vi "PostProcess.vi"(8 "error in (no error)":errorcluster, 10 "Variant in":variant, 11 "ONNX Angle Class in":refnum<class "ONNX Angle Class.lvclass">) -> (0 "error out":errorcluster, 2 "Variant out":variant, 3 "ONNX Angle Class out":refnum<class "ONNX Angle Class.lvclass">)   [LabVIEW 2017, in "ONNX Angle Class Library.lvlib" / "ONNX Angle Class.lvclass"]
uses:
  ONNX Angle Class.lvclass
  <vilib>/picture/picture.llb/imagedata.ctl
  ONNX Angle Class Library.lvlib
panel:
  out "image":picture
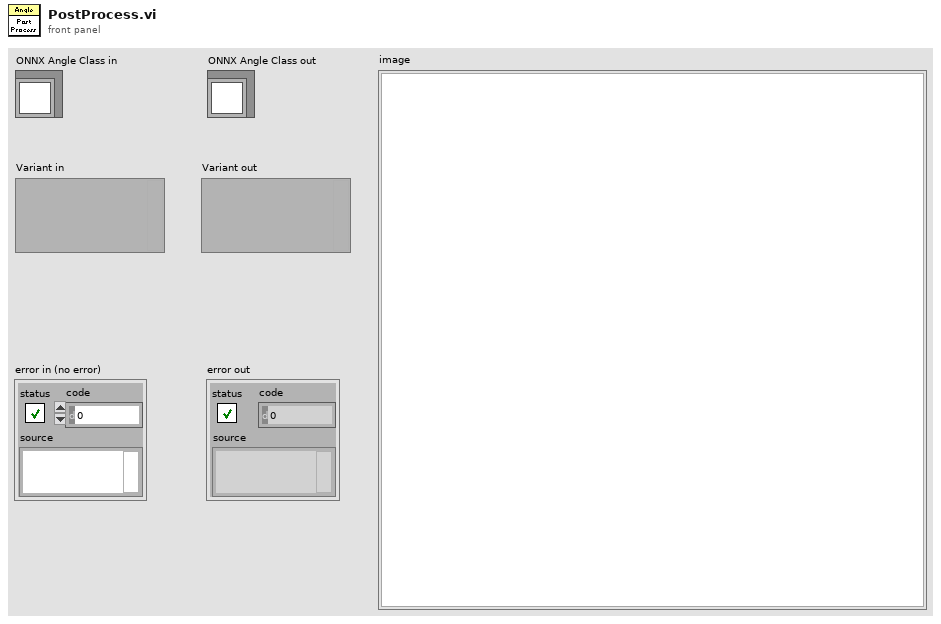
[diagram p1: front panel]
types:
  T1 = typedef "imagedata.ctl" = cluster{"image type":i32, "image depth":i32, "image":u8[], "mask":u8[], "colors":u32[], "Rectangle":cluster{"left":i16, "top":i16, "right":i16, "bottom":i16}}
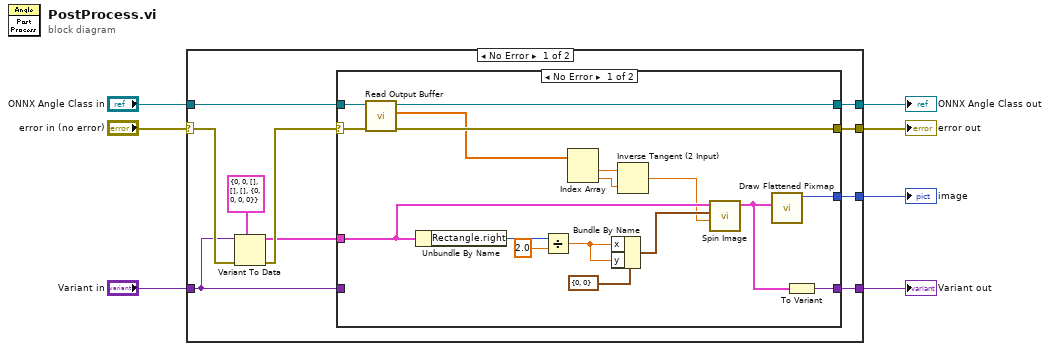
[diagram p0: block diagram]
diagram:
  n1 = case shown="No Error" "error in (no error)" {
    selector: "error in (no error)" -> [w16 w38]
    tunnel: "Variant in" -> [w12 w39]
    tunnel: "ONNX Angle Class in" -> [w15 w40]
    tunnel: [w14 w40] -> w6
    tunnel: [w11 w39] -> w2
    tunnel: [w13 w38] -> w3
    tunnel: [w8 _] -> w1
    frame No Error {
      n2 = Variant To Data(error in=w16, type=T1 {"image type"=0, "image depth"=0, "image"=[], "mask"=[], "colors"=[], "Rectangle"={"left"=0, "top"=0, "right"=0, "bottom"=0}} ("image data"), Variant=w12) -> (data=w9:T1, error out=w17:errorcluster)
      n3 = case shown="No Error" w17 {
        selector: w17 -> [w32 w36]
        tunnel: w15 -> [w33 w37]
        tunnel: [w31 w37] -> w14
        tunnel: [w30 w36] -> w13
        tunnel: w12 -> [_ w35]
        tunnel: [w34 w35] -> w11
        tunnel: w9 -> [w21 _]
        tunnel: [w19 _] -> w8
        frame No Error {
          n4 = call-dynamic "Read Output Buffer.vi"("error in (no error)"=w32, "ONNX Class in"=w33) -> ("error out"=w30:errorcluster, "Output Buffer"=w22:sgl[], "ONNX Class out"=w31:refnum<class "ONNX Angle Class.lvclass">)  [unwired: 7 in]
          n5 = Unbundle By Name(w21) -> ("Rectangle.right"=w27:i16)
          n6 = Divide(x=w27, y=2.0) -> (x/y=w26:dbl)
          n7 = Index Array(array=w22) -> (element #1=w29:sgl, element #2=w28:sgl)  [unwired: 2 in]
          n8 = Bundle By Name(cluster=cluster{"x":i16, "y":i16} {"x"=0, "y"=0} ("RotationPoint"), "x"=w26, "y"=w26) -> (w25:cluster{"x":i16, "y":i16})
          n9 = Inverse Tangent (2 Input)(1:w28, 2:w29) -> (0:w18:sgl)
          n10 = call "Spin Image.vi"("Angle [rad]"=w18, "RotationPoint"=w25, "Image In"=w21) -> ("Image Out"=w20:T1)  [unwired: 8 in]
          n11 = call <vilib>:"Draw Flattened Pixmap.vi"("image data"=w20) -> ("new picture"=w19:picture)  [unwired: 8 in]
          n12 = To Variant(anything=w20) -> (Variant=w34:variant)
        }
        frame Error {
        }
      }
    }
    frame Error {
    }
  }
  "error out" <- w3
  "ONNX Angle Class out" <- w6
  "Variant out" <- w2
  "image" <- w1
